vi "read_c_string_at_memory_address_to_file.vi"(6 "string_length":u64, 7 "File Path":path, 8 "error in (no error)":errorcluster, 11 "memory_address":u64) -> (0 "error out":errorcluster, 3 "memory_address out":u64)   [LabVIEW 2020, in "reqwest.lvlib"]
uses:
  reqwest.lvlib
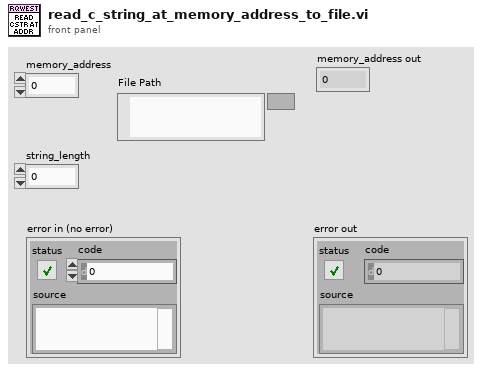
[diagram p1: front panel]
types:
  T1 = enum16{"open", "replace", "create", "open or create", "replace or create", "replace or create with confirmation"}
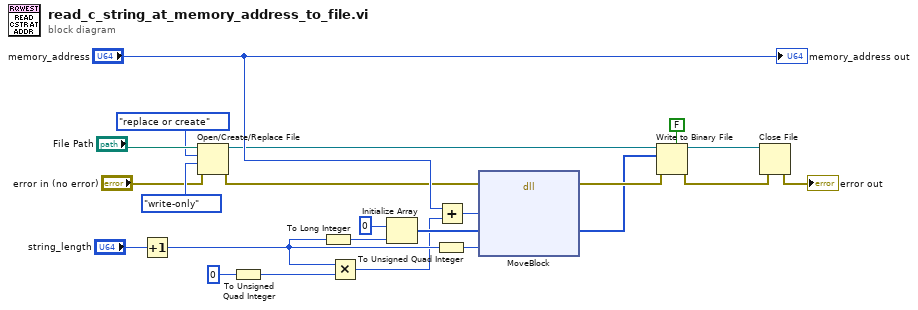
[diagram p0: block diagram]
diagram:
  n1 = Increment(x="string_length") -> (x+1=w21:u64)
  n2 = Open/Create/Replace File(file path (use dialog)="File Path", error in="error in (no error)", operation (0:open)=T1."replace or create", access (0:read/write)=enum16{"read/write", "read-only", "write-only"}."write-only") -> (refnum out=w19:refnum<file>, error out=w12:errorcluster)  [unwired: 2 in, 1 out]
  n3 = To Unsigned Quad Integer(1:u64 0 ("number")) -> (0:w5:u64)
  n4 = To Long Integer(number=w21) -> (32bit integer=w8:i32)
  n5 = Multiply(x=w21, y=w5) -> (x*y=w6:u64)
  n6 = Initialize Array(u8 0, w8) -> (w9:u8[])
  n7 = To Unsigned Quad Integer(1:w21) -> (0:w7:u64)
  n8 = Add(x="memory_address", y=w6) -> (x+y=w11:u64)
  n9 = dll-call lib="LabVIEW" fn="MoveBlock"(error in=w12, "src"=w11, "dst"=w9, "size"=w7) -> (error out=w3:errorcluster, "dst"=w2:u8[])  [unwired: 5 in, 1 out]
  n10 = Write to Binary File(file (use dialog)=w19, data=w2, error in=w3, 5:FALSE ("prepend array or string size? (T)")) -> (refnum out=w16:refnum<file>, error out=w15:errorcluster)  [unwired: 2 in, 1 out]
  n11 = Close File(refnum=w16, error in=w15) -> (error out=→"error out":errorcluster)  [unwired: 1 out]
  "memory_address out" <- "memory_address"
